vi "DMA Transfer Process.vi"(7 "Clock Domain":refnum<k21>="40 MHz Onboard Clock", 10 "Local":refnum<k21>, 11 "DMA":refnum<k21>) -> ()   [LabVIEW 2012]
uses:
  <vilib>/Platform/TimedLoop/XDataNode/wakeup.ctl
  <vilib>/Platform/TimedLoop/XDataNode/XDNodeRunTimeDep.lvlib
  <vilib>/Platform/TimedLoop/XDataNode/nitl_modes.ctl
  <vilib>/Platform/TimedLoop/XDataNode/timing_clust.ctl
  <vilib>/Platform/TimedLoop/XDataNode/XDataNode.xnode
  <vilib>/rvi/DataTransferAndStorage/Container/XNode/niFpgaContainer.xnode
  <vilib>/rvi/FIFO/Fifo_Resource/niFpgaFifoEmulationRefIn.vi
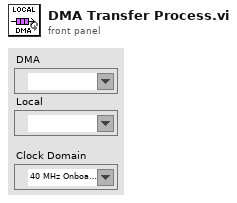
[diagram p1: front panel]
types:
  T1 = typedef "XDNodeRunTimeDep.lvlib/timing_clust.ctl" = cluster{"Expected End [f-1]":u64, "Actual End [f-1]":u64, "Finished Late? [f-1]":bool, "Expected End [i-1]":u64, "Actual End [i-1]":u64, "Finished Late? [i-1]":bool, "Expected Start [i]":u64, "Actual Start [i]":u64, "Expected Start [f]":u64, "Actual Start [f]":u64, "Source Name":string, "Structure Name":string, "Period":i64, "Deadline":i64, "Offset":i64, "Start":i64, "Priority":i32, "Timeout":i32, "Mode":T2, "Wakeup Reason":T3, "Error":errorcluster, "Source Type":string, "Secondary Source Type":string, "Global End Time":u64, "Global Start Time":u64, "Frame Duration":u64, "Iteration Duration":u64, "Assigned CPU":i32, "I/O Scan Engine Mode":u32}
  T2 = typedef "XDNodeRunTimeDep.lvlib/nitl_modes.ctl" = enum32{"No Change", "Process missed periods, maintain original phase", "Discard missed periods, maintain original phase", "Process missed periods, ignore original phase", "Discard missed periods, ignore original phase"}
  T3 = typedef "XDNodeRunTimeDep.lvlib/wakeup.ctl" = enum32{"Normal", "Aborted", "Asynchronous wakeup", "Timing source error", "Timed loop error", "Timeout"}
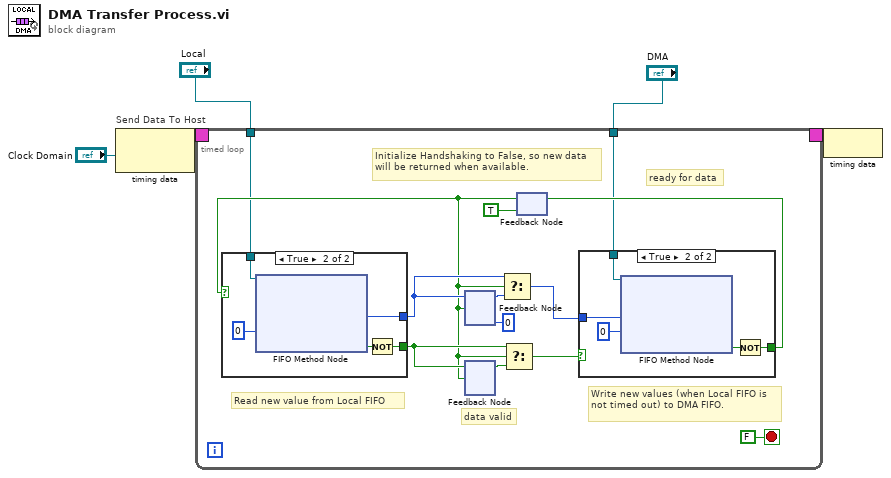
[diagram p0: block diagram]
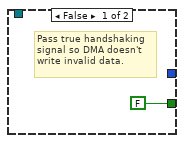
[diagram p2: hidden frame]
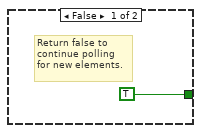
[diagram p3: hidden frame]
diagram:
  n1 = node-c288("Clock Domain") -> (w5:T1)
  n2 = timed-loop "Send Data To Host" {
    timing: w5 -> [_]
    timing-out: [_] -> w4
    tunnel: "DMA" -> [w7]
    tunnel: "Local" -> [w6]
    stop <- FALSE stop-if-true
    # "Read new value from Local FIFO"
    # "ready for data"
    # "data valid"
    # "Initialize Handshaking to False, so new data will be returned when available."
    # "Write new values (when Local FIFO is not timed out) to DMA FIFO."
    n3 = feedback #1(i16 0 ("Element")) -> (w14:i16)
    n4 = feedback #2() -> (w10:bool)  [unwired: 1 in]
    n5 = feedback #3(TRUE ("Timed Out?")) -> (w9:bool)
    n6 = case shown="True" w9 {
      tunnel: [FALSE ("Timed Out?") w24] -> w11
      tunnel: [_ w21] -> w13
      tunnel: w6 -> [_ w20]
      frame False {
        # "Pass true handshaking\nsignal so DMA doesn't\nwrite invalid data."
      }
      frame True {
        n7 = xnode ("FIFO Method Node")("Timeout"=0, "FIFO In"=w20) -> ("Element"=w21:i16, "Timed Out?"=w23:bool)  [unwired: 1 out]
        n8 = Not(x=w23) -> (.not. x?=w24:bool)
      }
    }
    n9 = feedback-in #1(w13, w9) -> ()
    n10 = feedback-in #2(w11, w9) -> ()
    n11 = Select(t=w13, s=w9, f=w14) -> (s? t:f=w15:i16)
    n12 = Select(t=w11, s=w9, f=w10) -> (s? t:f=w8:bool)
    n13 = case shown="True" w8 {
      tunnel: [TRUE ("Timed Out?") w30] -> w16
      tunnel: w15 -> [_ w29]
      tunnel: w7 -> [_ w26]
      frame False {
        # "Return false to \ncontinue polling\nfor new elements."
      }
      frame True {
        n14 = xnode ("FIFO Method Node")("Element"=w29, "Timeout"=0, "FIFO In"=w26) -> ("Timed Out?"=w27:bool)  [unwired: 1 out]
        n15 = Not(x=w27) -> (.not. x?=w30:bool)
      }
    }
    n16 = feedback-in #3(w16) -> ()
  }
  n17 = node-c288(w4) -> ()
